vi "queryModel (SubVI).vi"(2 "errorIn":errorcluster, 3 "queryInStr":string, 4 "queryModel":refnum<vi>) -> (0 "errorOut":errorcluster, 1 "queryOutStr":string)   [LabVIEW 2010]
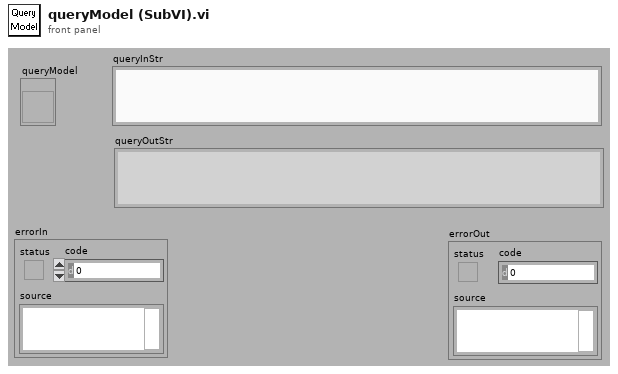
[diagram p1: front panel]
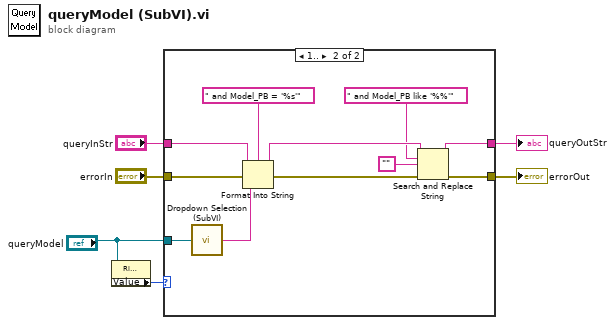
[diagram p0: block diagram]
diagram:
  n1 = property on="Property Node" class="Ring (strict)"(reference="queryModel") -> ("Value"=w2:u16)  [unwired: 1 in, 2 out]
  n2 = case shown="1.." w2 {
    tunnel: "queryModel" -> [_ w19]
    tunnel: [w8 w11] -> w5
    tunnel: [w7 w10] -> w6
    tunnel: "errorIn" -> [w7 w18]
    tunnel: "queryInStr" -> [w8 w17]
    frame 0, Default {
    }
    frame 1.. {
      n3 = call "Dropdown Selection (SubVI).vi"("reference"=w19) -> ("element"=w9:string)
      n4 = Format Into String(format string=" and Model_PB = '%s'", initial string=w17, error in=w18, w9) -> (resulting string=w15:string, error out=w14:errorcluster)
      n5 = Search and Replace String(input string=w15, search string=" and Model_PB like '%%'", replace string="" ("replace string (\"\")"), error in=w14) -> (result string=w11:string, error out=w10:errorcluster)  [unwired: 6 out]
    }
  }
  "errorOut" <- w6
  "queryOutStr" <- w5
